vi "Health_accel.vi"(5 "LIMITE MIN":dbl, 6 "LIMITE MAX":dbl, 7 "Aceleraciones":dbl[][](array[numeric])) -> (0 "concatenated string":string, 1 "ACELEROMETROS OK":bool)   [LabVIEW 2015]
panel:
  out "BAJA SEÑAL":bool
  out "ACEL.SATURADO":bool
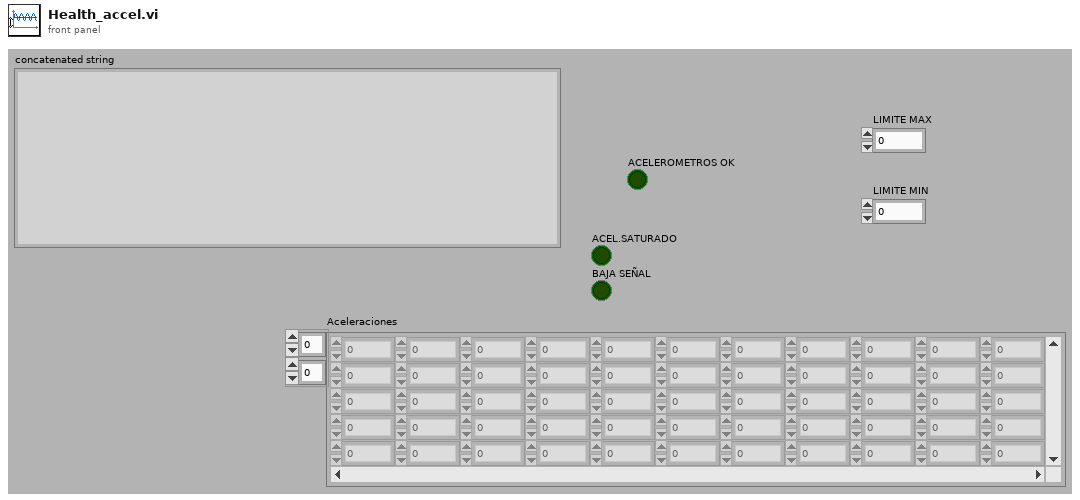
[diagram p1: front panel]
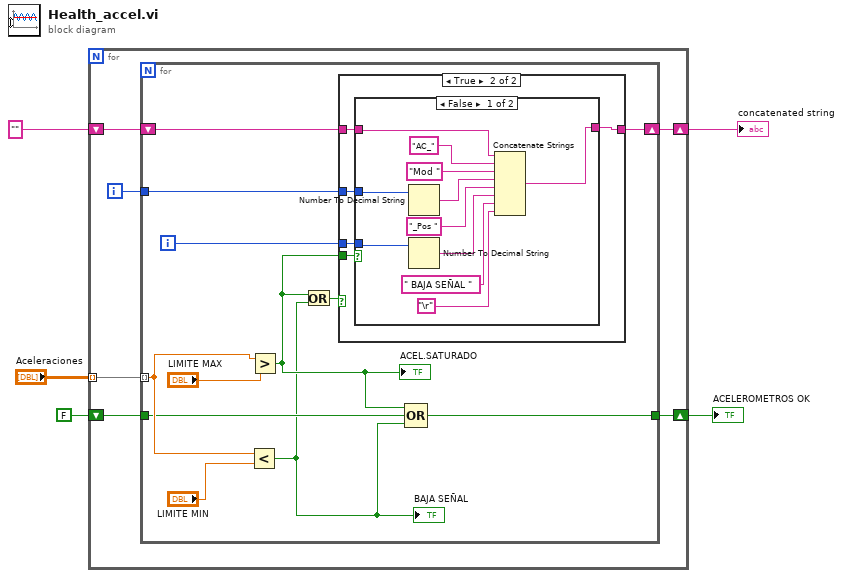
[diagram p0: block diagram]
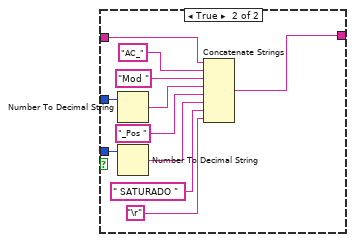
[diagram p3: hidden frame]
diagram:
  n1 = for {
    tunnel: "Aceleraciones" -> [w11] mode=indexing
    shift-right: [w9] -> w3
    shift-left: "" -> [w10]
    shift-right: [w6] -> w1
    shift-left: FALSE -> [w7]
    i -> [w8]
    n2 = for {
      tunnel: w11 -> [w21] mode=indexing
      shift-right: [w18] -> w9
      shift-left: w10 -> [w19]
      tunnel: w8 -> [w17]
      tunnel: w7 -> [w14]
      tunnel: [w12] -> w6
      i -> [w16]
      n3 = Less?(x=w21, y="LIMITE MIN") -> (x < y?=w13:bool)
      "BAJA SEÑAL" <- w13
      n4 = Greater?(x=w21, y="LIMITE MAX") -> (0:w15:bool)
      "ACEL.SATURADO" <- w15
      n5 = Or(x=w15, y=w13) -> (x .or. y?=w20:bool)
      n6 = case shown="True" w20 {
        tunnel: w15 -> [_ w29]
        tunnel: w19 -> [w24 w28]
        tunnel: [w24 w25] -> w18
        tunnel: w17 -> [_ w27]
        tunnel: w16 -> [_ w26]
        frame False {
        }
        frame True {
          n7 = case shown="False" w29 {
            tunnel: w28 -> [w33 w44]
            tunnel: w27 -> [w31 w51]
            tunnel: w26 -> [w30 w50]
            tunnel: [w32 w43] -> w25
            frame False {
              n8 = Number To Decimal String(number=w31) -> (decimal integer string=w38:string)  [unwired: 1 in]
              n9 = Number To Decimal String(number=w30) -> (decimal integer string=w36:string)  [unwired: 1 in]
              n10 = Concatenate Strings(w33, "AC_", "Mod ", w38, "_Pos ", w36, " BAJA SEÑAL ", "\r") -> (w32:string)
            }
            frame True {
              n11 = Number To Decimal String(number=w51) -> (decimal integer string=w47:string)  [unwired: 1 in]
              n12 = Number To Decimal String(number=w50) -> (decimal integer string=w45:string)  [unwired: 1 in]
              n13 = Concatenate Strings(w44, "AC_", "Mod ", w47, "_Pos ", w45, " SATURADO ", "\r") -> (w43:string)
            }
          }
        }
      }
      n14 = Compound Arithmetic op=OR(w15, w14, w13) -> (w12:bool)
    }
  }
  "ACELEROMETROS OK" <- w1
  "concatenated string" <- w3
